vi "Create DataColumns.vi"(8 "错误输入（无错误）":errorcluster, 10 "DataType":variant[](array[variant]), 11 "ColumnName Array":string[](array[string])) -> (0 "错误输出":errorcluster, 3 "DataColumns":refnum<k24>[](array[refnum]))   [LabVIEW 2012, in "DataGridView.lvlib"]
uses:
  DataGridView.lvlib
  System.Data
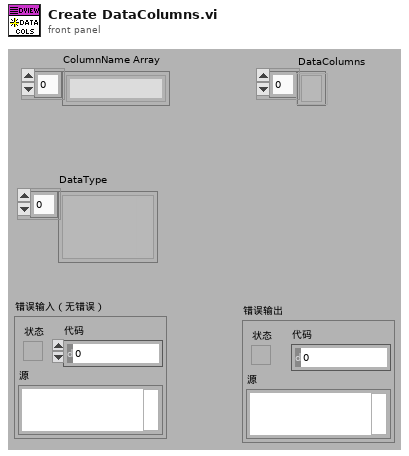
[diagram p1: front panel]
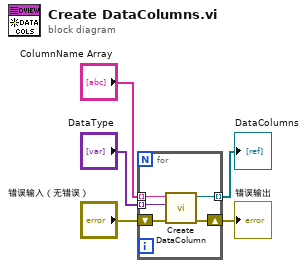
[diagram p0: block diagram]
diagram:
  n1 = for {
    shift-right: [w9] -> w4
    shift-left: "错误输入（无错误）" -> [w10]
    tunnel: "ColumnName Array" -> [w8] mode=indexing
    tunnel: "DataType" -> [w7] mode=indexing
    tunnel: [w6] -> w1 mode=indexing
    n2 = call "Create DataColumn.vi"("错误输入（无错误）"=w10, "DataType"=w7, "columnName"=w8) -> ("错误输出"=w9:errorcluster, "DataColumn"=w6:refnum<k24>)  [unwired: 7 in]
  }
  "错误输出" <- w4
  "DataColumns" <- w1
